vi "FTW-SQLite-Backup-Worker.vi"(0 "Event Ref":refnum<user-event>, 1 "Backup Object":u64 format="%016x", 2 "Destination Database Filepath":path, 3 "SQLite Connector":refnum<class "FTW-SQLite-Connector.lvclass">) -> ()   [LabVIEW 2013, in "FTW-SQLite-Connector.lvclass"]
uses:
  FTW-SQLite-Connector.lvclass
  FTW-SQLite-AsyncOperation.ctl
panel:
  # "Inputs"
  # "Outputs"
  # "This async worker has no outputs."
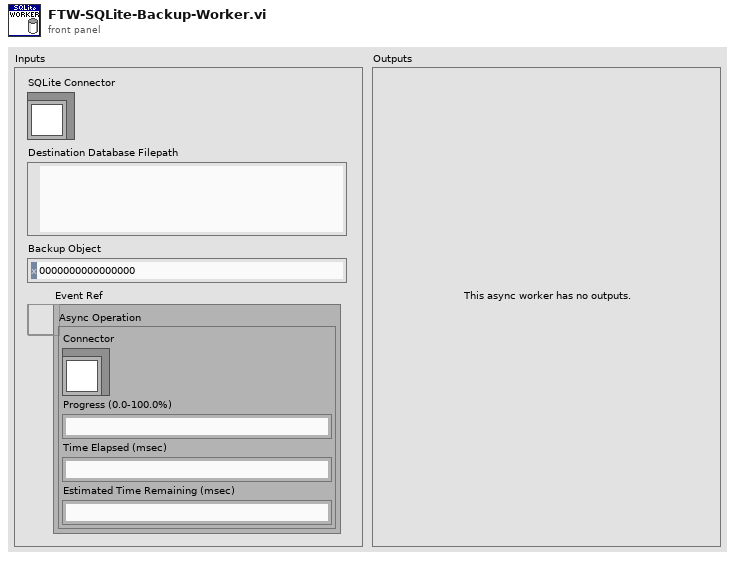
[diagram p1: front panel]
types:
  T1 = typedef "FTW-SQLite-Connector.lvclass/FTW-SQLite-AsyncOperation.ctl" = cluster{"Connector":refnum<class "FTW-SQLite-Connector.lvclass">, "Progress (0.0-100.0%)":dbl, "Time Elapsed (msec)":u32, "Estimated Time Remaining (msec)":u32}
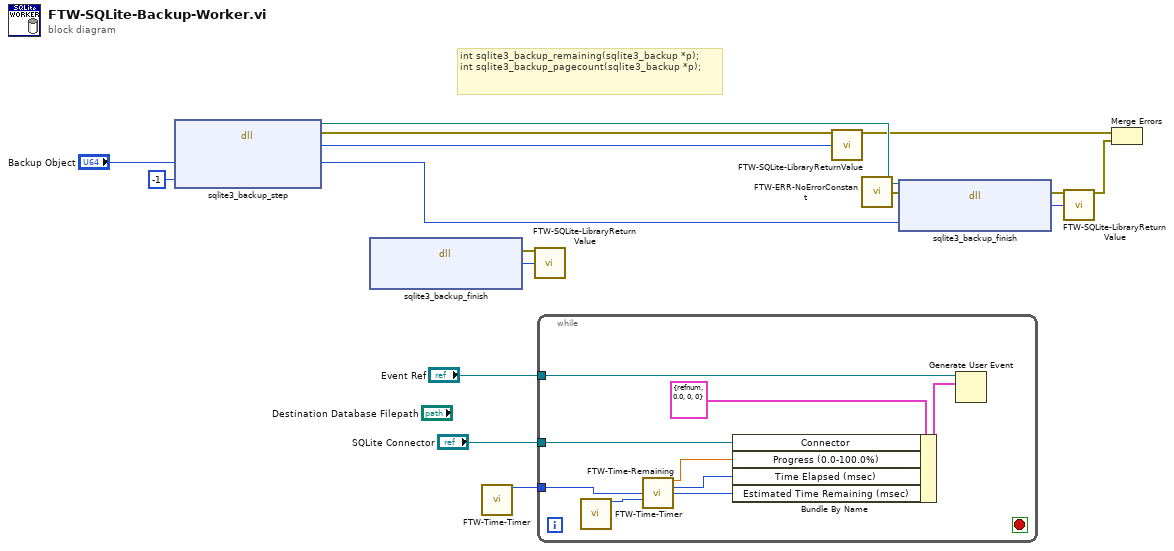
[diagram p0: block diagram]
diagram:
  # "int sqlite3_backup_remaining(sqlite3_backup *p);\nint sqlite3_backup_pagecount(sqlite3_backup *p);"
  n1 = dll-call lib="?" fn="sqlite3_backup_step"("Backup Object"="Backup Object", "NumPages"=-1) -> (path out=w13:path, error out=w11:errorcluster, "Return Type"=w9:i32, "Backup Object"=w16:u64)  [unwired: 4 in]
  n2 = dll-call lib="?" fn="sqlite3_backup_finish"() -> (error out=w2:errorcluster, "Return Value"=w3:i32)  [unwired: 5 in, 1 out]
  n3 = call "FTW-Time-Timer.vi"() -> ("Current Tick Count"=w1:u32)  [unwired: 13 in, 2 out]
  n4 = call "FTW-SQLite-LibraryReturnValue.vi"("error in"=w2, "Return Value"=w3) -> ()  [unwired: 13 in, 1 out]
  n5 = while {
    tunnel: "Event Ref" -> [w25]
    tunnel: "SQLite Connector" -> [w22]
    tunnel: w1 -> [w20]
    stop <- _ stop-if-true
    n6 = call "FTW-Time-Timer.vi"() -> ("Current Tick Count"=w21:u32)  [unwired: 13 in, 2 out]
    n7 = call "FTW-Time-Remaining.vi"("Initial Timestamp"=w20, "Current Timestamp"=w21) -> ("Percent Done (0.0-100.0%)"=w19:dbl, "Time Elapsed (msec)"=w18:u32, "Estimated Time Remaining (msec)"=w17:u32)  [unwired: 9 in, 2 out]
    n8 = Bundle By Name(cluster=T1 {"Connector"=refnum, "Progress (0.0-100.0%)"=0.0, "Time Elapsed (msec)"=0, "Estimated Time Remaining (msec)"=0} ("event data"), "Connector"=w22, "Progress (0.0-100.0%)"=w19, "Time Elapsed (msec)"=w18, "Estimated Time Remaining (msec)"=w17) -> (w23:T1)
    n9 = Generate User Event(user event=w25, event data cluster=w23) -> ()  [unwired: 2 in, 2 out]
  }
  n10 = call "FTW-SQLite-LibraryReturnValue.vi"("error in"=w11, "Return Value"=w9) -> ("error out"=w10:errorcluster)  [unwired: 13 in]
  n11 = call "FTW-ERR-NoErrorConstant.vi"() -> ("no error"=w8:errorcluster)
  n12 = dll-call lib="?" fn="sqlite3_backup_finish"(path in=w13, error in=w8, "Backup Object"=w16) -> (error out=w15:errorcluster, "Return Value"=w14:i32)  [unwired: 2 in, 1 out]
  n13 = call "FTW-SQLite-LibraryReturnValue.vi"("error in"=w15, "Return Value"=w14) -> ("error out"=w12:errorcluster)  [unwired: 13 in]
  n14 = Merge Errors(w10, w12) -> ()  [unwired: 1 out]
